vi "CreateScreenShot.vi"(8 "error in (no error)":errorcluster, 9 "Screenshot name":string, 10 "base path":path, 11 "reference":refnum<vi>) -> (0 "error out":errorcluster)   [LabVIEW 2018]
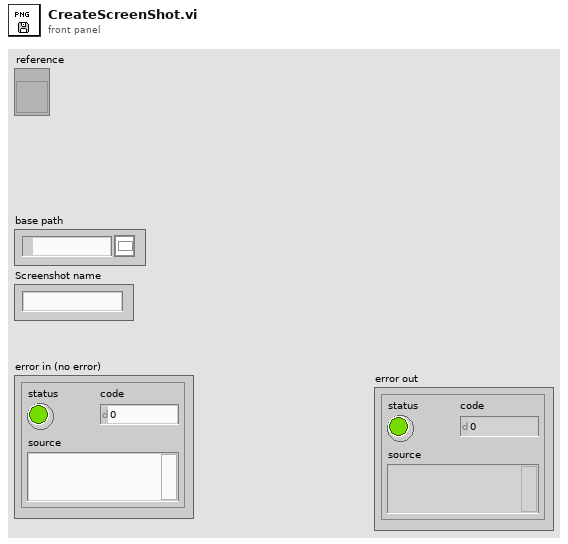
[diagram p1: front panel]
types:
  T1 = typedef "imagedata.ctl" = cluster{"image type":i32, "image depth":i32, "image":u8[], "mask":u8[], "colors":u32[], "Rectangle":cluster{"left":i16, "top":i16, "right":i16, "bottom":i16}}
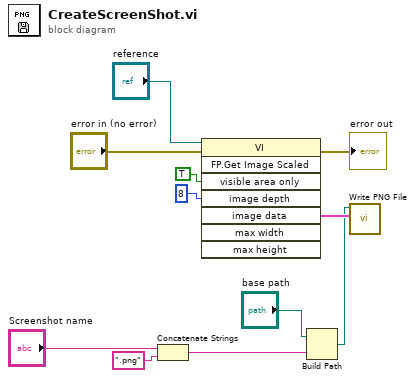
[diagram p0: block diagram]
diagram:
  n1 = Concatenate Strings("Screenshot name", ".png" ("string")) -> (w7:string)
  n2 = invoke class="VI" method="FP.Get Image Scaled"(reference="reference", error in="error in (no error)", "visible area only"=TRUE ("Visible Area Only"), "image depth"=8 ("Image Depth")) -> (error out=→"error out":errorcluster, "image data"=w9:T1)  [unwired: 4 in, 6 out]
  n3 = Build Path(base path="base path", name or relative path=w7) -> (appended path=w8:path)
  n4 = call <vilib>:"Write PNG File.vi"("image data"=w9, "path to PNG file"=w8) -> ()  [unwired: 8 in, 2 out]
